vi "EnableBroadcasting.vi"(8 "error in (no error)":errorcluster, 10 "Broadcasting":T1, 11 "SM1000-control in":T2) -> (0 "error out":errorcluster, 3 "SM1000-control out":T2)   [LabVIEW 2013, in "SLMControl.lvlib" / "SM1000.lvclass"]
doc: "Enables/disables the broadcast function of the EC1000.\n\nThe host must have exclusive control of the EC1000 ('TakeHostControl') before using this command.\n\nCommand: <\"TakeHostControl\" or 2>,<0 == disable, 1 == enable>\nReturns: \"0\""
uses:
  SM1000.lvclass
  Object-reference.ctl
  Broadcasting.ctl
  SM1000.lvclass/SM1000.ctl
  Custom-errors.ctl
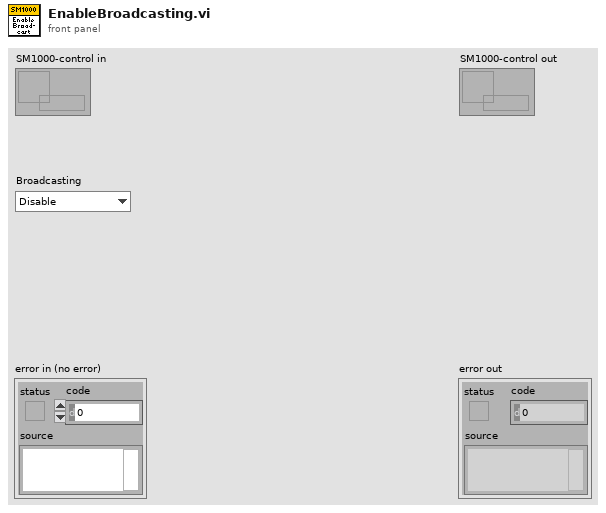
[diagram p1: front panel]
types:
  T1 = typedef "SLMControl.lvlib/SM1000.lvclass/Broadcasting.ctl" = enum16{"Disable", "Enable"}
  T2 = typedef "SLMControl.lvlib/SM1000.lvclass/Object-reference.ctl" = refnum<data-value>
  T3 = typedef "SLMControl.lvlib/SM1000.lvclass/Custom-errors.ctl" = enum16{"No error", "Not implemented", "Command not recognized", "Invalid input", "No connection", "Timeout", "Resource not loaded"}
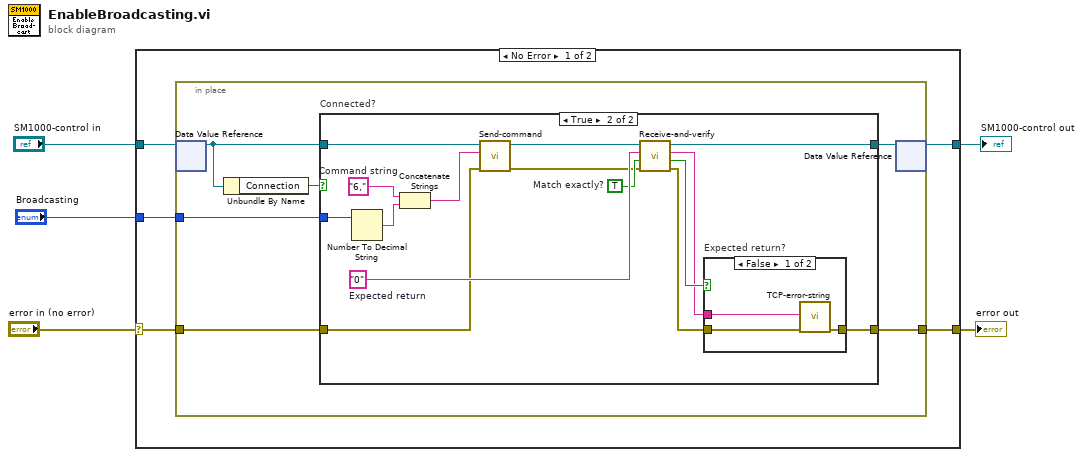
[diagram p0: block diagram]
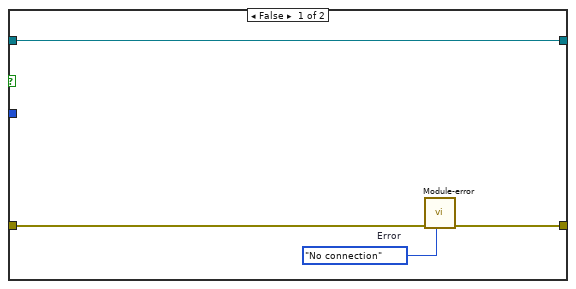
[diagram p2: hidden frame]
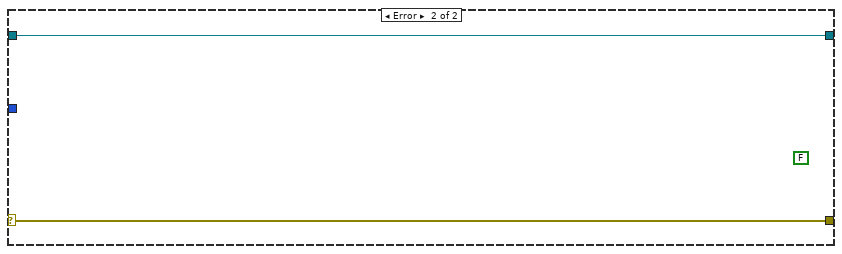
[diagram p4: hidden frame]
diagram:
  n1 = case shown="No Error" "error in (no error)" {
    selector: "error in (no error)" -> [w8 w41]
    tunnel: [w7 w41] -> w4
    tunnel: [w9 w40] -> w2
    tunnel: "SM1000-control in" -> [w10 w40]
    tunnel: "Broadcasting" -> [w6 _]
    frame No Error {
      n2 = in-place {
        in-place-border: w8 -> [w16]
        in-place-border: [w13] -> w7
        in-place-border: w6 -> [w11]
        n3 = in-place-dvr #1(w10) -> (w14:refnum<class "SM1000.lvclass">)  [unwired: 1 out]
        n4 = Unbundle By Name(w14) -> ("Connection"=w15:bool)
        n5 = case "Connected?" shown="True" w15 {
          tunnel: w16 -> [w20 w28]
          tunnel: w14 -> [w18 w35]
          tunnel: [w19 w26] -> w13
          tunnel: [w18 w25] -> w12
          tunnel: w11 -> [_ w24]
          frame False {
            w17 = Custom-errors."No connection"  # Error
            n6 = call "Module-error.vi"("Error"=w17, "error in (no error)"=w20) -> ("error out"=w19:errorcluster)  [unwired: 9 in]
          }
          frame True {
            w32 = TRUE  # Match exactly?
            w33 = "0"  # Expected return
            w22 = "6,"  # Command string
            n7 = Number To Decimal String(number=w24) -> (decimal integer string=w23:string)  [unwired: 1 in]
            n8 = Concatenate Strings(w22, w23) -> (w21:string)
            n9 = call "Send-command.vi"("error in (no error)"=w28, "Command string"=w21, "SM1000-control in"=w35) -> ("error out"=w31:errorcluster, "SM1000-control out"=w34:refnum<class "SM1000.lvclass">)  [unwired: 7 in]
            n10 = call "Receive-and-verify.vi"("error in (no error)"=w31, "Match exactly?"=w32, "Expected return string"=w33, "SM1000-control in"=w34) -> ("error out"=w27:errorcluster, "Verified?"=w30:bool, "Return string"=w29:string, "SM1000-control out"=w25:refnum<class "SM1000.lvclass">)  [unwired: 4 in]
            n11 = case "Expected return?" shown="False" w30 {
              tunnel: w29 -> [w38 _]
              tunnel: w27 -> [w37 w39]
              tunnel: [w36 w39] -> w26
              frame False {
                n12 = call "TCP-error-string.vi"("error in (no error)"=w37, "Retun code"=w38) -> ("error out"=w36:errorcluster)  [unwired: 9 in]
              }
              frame True {
              }
            }
          }
        }
        n13 = in-place-dvr #1(w12) -> (w9:T2)  [unwired: 1 out]
      }
    }
    frame Error {
      (unwired) FALSE
    }
  }
  "error out" <- w4
  "SM1000-control out" <- w2
